vi "Test_ReadValue_NeverWritten_TimeoutError.vi"(8 "error in (no error)":errorcluster, 11 "TestCase in":refnum<class "TestQueueTransport.lvclass">) -> (0 "error out":errorcluster, 3 "TestCase out":refnum<class "TestQueueTransport.lvclass">)   [LabVIEW 2017, in "TestQueueTransport.lvclass"]
uses:
  TestQueueTransport.lvclass
  Source/Concrete/QueueTransport/QueueTransport.lvclass/QueueTransport.ctl
  <vilib>/Utility/error.llb/Error Cluster From Error Code.vi
  Source/Concrete/QueueTransport/QueueTransport.lvclass
panel:
  out "Return Error":errorcluster
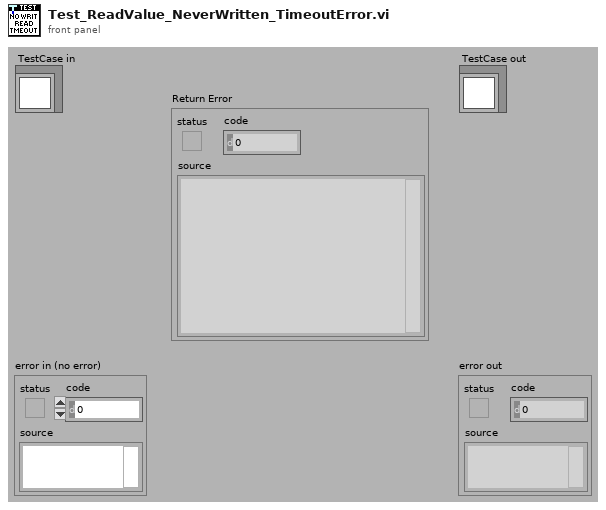
[diagram p1: front panel]
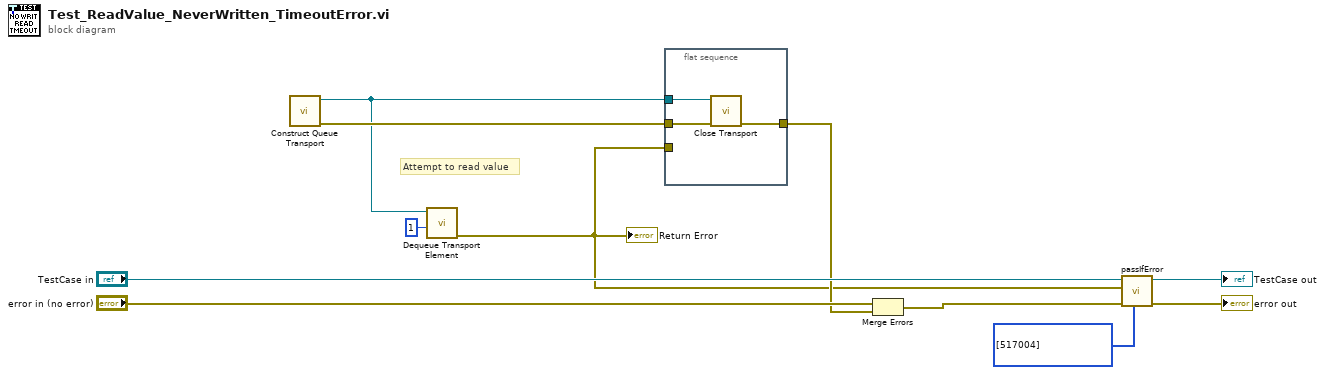
[diagram p0: block diagram]
diagram:
  # "Attempt to read value"
  n1 = call "Construct Queue Transport.vi"() -> ("error out"=w4:errorcluster, "QueueTransport"=w2:refnum<class "QueueTransport.lvclass">)  [unwired: 10 in]
  n2 = call "Dequeue Transport Element.vi"("Timeout In ms (-1)"=1, "QueueTransport"=w2) -> ("error out"=w1:errorcluster)  [unwired: 6 in, 3 out]
  "Return Error" <- w1
  n3 = flat-sequence {
    tunnel: w4 -> [w14]
    tunnel: [w13] -> w3
    tunnel: w2 -> [w12]
    tunnel: w1 -> [_]
    frame #0 {
      n4 = call-dynamic "Close Transport.vi"("error in (no error)"=w14, "QueueTransport"=w12) -> ("error out"=w13:errorcluster)  [unwired: 9 in]
    }
  }
  n5 = Merge Errors("error in (no error)", w3) -> (w6:errorcluster)
  n6 = call-dynamic "passIfError.vi"("passing error codes (default = any error code)"=i32[] [517004], "error in (no error)"=w6, "error"=w1, "TestCase in"="TestCase in") -> ("error out"=→"error out":errorcluster, "TestCase out"=→"TestCase out":refnum<class "TestQueueTransport.lvclass">)  [unwired: 6 in]
